vi "Main UI.vi"() -> ()   [LabVIEW 2011]
doc: "This template is for the Queued Message Handler design pattern.\n\nThe Event Handling Loop generates messages based on user interface actions.\n\nThe Message Handling Loop processes messages generated by the Event Handling Loop, or by other messages. The messages are string values, so new messages can be added easily to the Message Cases case structure in the Message Handling Loop. Each message cluster can also provide an optional value for Message Data, which is a variant that can be converted to whatever message-specific data is required."
uses:
  controls/UI Data.ctl
  support/Message Queue/Message Queue.lvlib
  support/User Event - Stop/User Event - Stop.lvlib
panel:
  out "DNL_Data Display <Replace Me>":string
  in  "DNL_Do Something Else <Replace Me>":bool
  in  "DNL_Do Something <Replace Me>":bool
  in  "DNL_Stop Button":bool
  # "These controls have associated \"Value Changed\" events configured in the Event Structure on the diagram.\n\nReplace them (and reconfigure the Event Structure) with the controls you need for your application."
  # "This template is for the Queued Message Handler design pattern.\n\nSee the block diagram for more information on how to use this template."
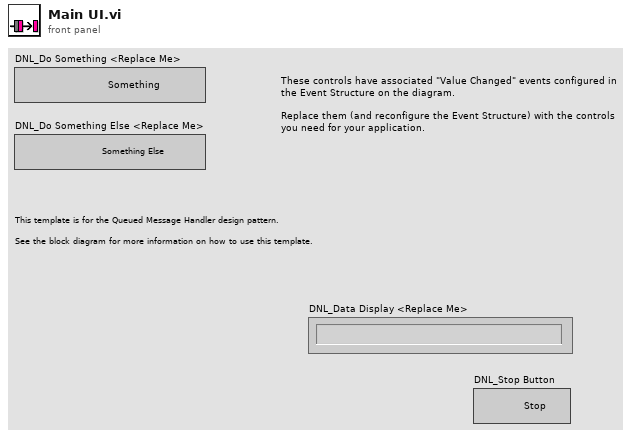
[diagram p1: front panel]
types:
  T1 = typedef "UI Data.ctl" = cluster{"DNL_Boolean <Replace Me>":bool, "DNL_String <Replace Me>":string, "DNL_Numeric <Replace Me>":dbl}
  T2 = typedef "Message Queue.lvlib/All Message Queues.ctl" = cluster{"DNL_UI":refnum<queue>}
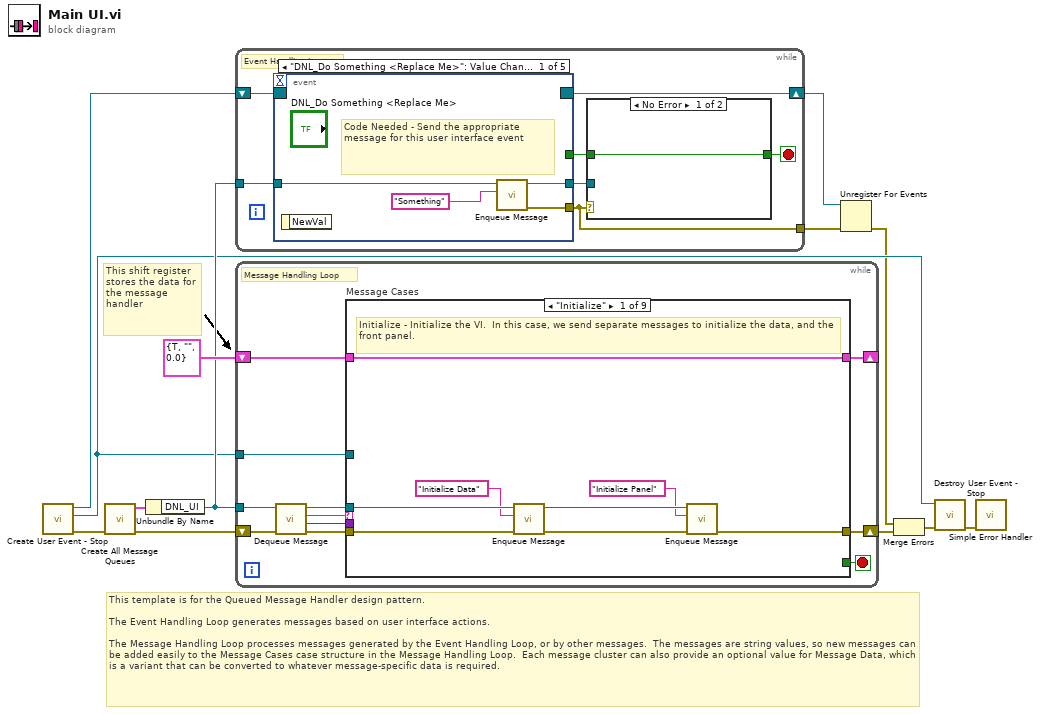
[diagram p0: block diagram]
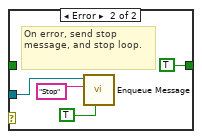
[diagram p2: hidden frame]
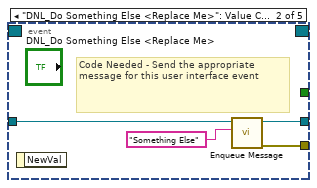
[diagram p3: hidden frame]
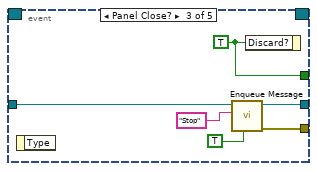
[diagram p4: hidden frame]
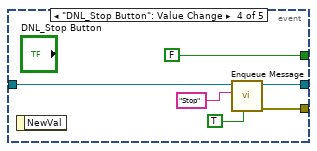
[diagram p5: hidden frame]
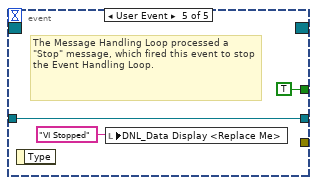
[diagram p6: hidden frame]
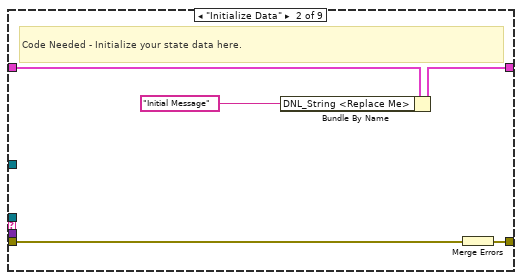
[diagram p7: hidden frame]
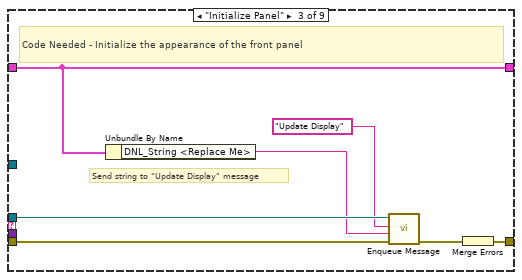
[diagram p8: hidden frame]
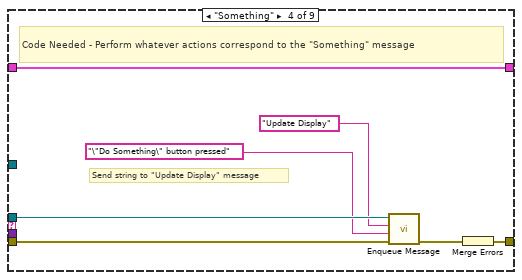
[diagram p9: hidden frame]
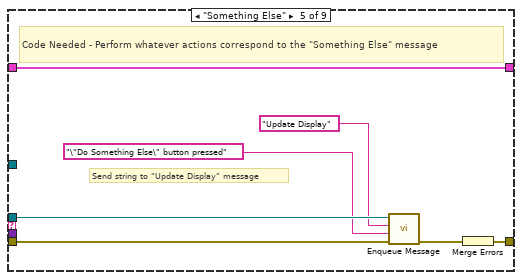
[diagram p10: hidden frame]
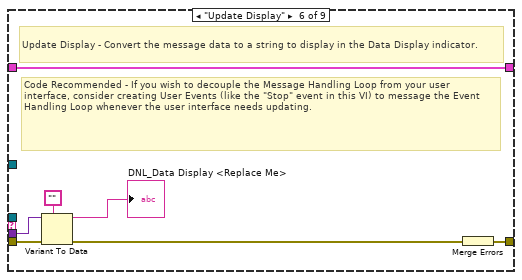
[diagram p11: hidden frame]
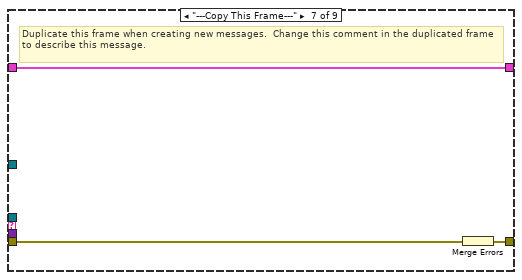
[diagram p12: hidden frame]
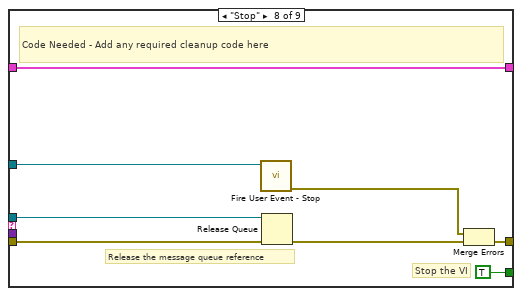
[diagram p13: hidden frame]
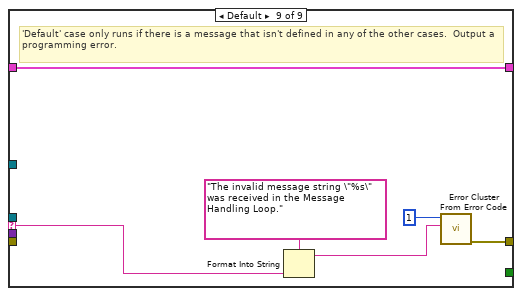
[diagram p14: hidden frame]
diagram:
  # "This template is for the Queued Message Handler design pattern.\n\nThe Event Handling Loop generates messages based on user interface actions.\n\nThe Message Handling Loop processes messages generated by the Event Handling Loop, or by other messages.  The messages are string values, so new messages can be added easily to the Message Cases case structure in the Message Handling Loop.  Each message cluster can also provide an optional value for Message Data, which is a variant that can be converted to whatever message-specific data is required."
  # "This shift register\nstores the data for the message handler"
  n1 = call "Create User Event - Stop.vi"() -> ("error out"=w7:errorcluster, "DNL_User Event - Stop"=w4:refnum<user-event>, "DNL_Stop Event Registration Refnum"=w8:refnum<event-registration>)  [unwired: 9 in]
  n2 = call "Create All Message Queues.vi"("error in (no error)"=w7) -> ("error out"=w13:errorcluster, "DNL_Message Queues out"=w11:T2)  [unwired: 9 in]
  n3 = Unbundle By Name(w11) -> ("DNL_UI"=w9:refnum<queue>)
  n4 = while {
    tunnel: w9 -> [w20]
    tunnel: [w16] -> w2
    shift-right: [w14] -> w1
    shift-left: w8 -> [w15]
    stop <- w18 stop-if-true
    # "Event Handling Loop"
    n5 = event shown="[0] \"DNL_Do Something <Replace Me>\": Value Change" {
      selector: w15 -> [_ _ _ _ _]
      dyn-events: [_ _ _ _ _] -> w14
      timeout: _ -> [_ _ _ _ _]
      tunnel: [_ _ w39 FALSE ("Discard?") TRUE ("Discard?")] -> w19
      tunnel: w20 -> [w29 w33 w38 w45 w48]
      tunnel: [w28 w31 w37 w44 _] -> w16
      tunnel: [w27 w32 w36 w42 w48] -> w17
      event "DNL_Do Something <Replace Me>": Value Change {
        # "Code Needed - Send the appropriate message for this user interface event"
        n6 = event-data() -> ()  [unwired: 1 in, 1 out]
        n7 = call "Enqueue Message.vi"("DNL_Message"="Something" ("Message"), "DNL_Message Queue"=w29) -> ("error out"=w28:errorcluster, "DNL_dup Message Queue"=w27:refnum<queue>)  [unwired: 8 in]
      }
      event "DNL_Do Something Else <Replace Me>": Value Change {
        # "Code Needed - Send the appropriate message for this user interface event"
        n8 = event-data() -> ()  [unwired: 1 in, 1 out]
        n9 = call "Enqueue Message.vi"("DNL_Message"="Something Else" ("Message"), "DNL_Message Queue"=w33) -> ("error out"=w31:errorcluster, "DNL_dup Message Queue"=w32:refnum<queue>)  [unwired: 8 in]
      }
      event Panel Close? {
        w39 = TRUE ("Discard?")
        n10 = event-data() -> ()  [unwired: 1 in, 1 out]
        n11 = call "Enqueue Message.vi"("DNL_Priority Message? (F)"=TRUE ("Priority Message? (F)"), "DNL_Message"="Stop" ("Message"), "DNL_Message Queue"=w38) -> ("error out"=w37:errorcluster, "DNL_dup Message Queue"=w36:refnum<queue>)  [unwired: 7 in]
        n12 = event-data("Discard?"=w39) -> ()  [unwired: 1 in, 1 out]
      }
      event "DNL_Stop Button": Value Change {
        n13 = event-data() -> ()  [unwired: 1 in, 1 out]
        n14 = call "Enqueue Message.vi"("DNL_Priority Message? (F)"=TRUE ("Priority Message? (F)"), "DNL_Message"="Stop" ("Message"), "DNL_Message Queue"=w45) -> ("error out"=w44:errorcluster, "DNL_dup Message Queue"=w42:refnum<queue>)  [unwired: 7 in]
      }
      event User Event {
        # "The Message Handling Loop processed a \"Stop\" message, which fired this event to stop the Event Handling Loop."
        n15 = event-data() -> ()  [unwired: 1 in, 1 out]
        n16 = local write "DNL_Data Display <Replace Me>"("VI Stopped" ("VI Stopped")) -> ()
      }
    }
    n17 = case shown="No Error" w16 {
      tunnel: [w21 TRUE ("Discard?")] -> w18
      tunnel: w19 -> [w21 _]
      tunnel: w17 -> [_ w24]
      frame No Error {
      }
      frame Error {
        # "On error, send stop message, and stop loop."
        n18 = call "Enqueue Message.vi"("DNL_Priority Message? (F)"=TRUE ("Priority Message? (F)"), "DNL_Message"="Stop" ("Message"), "DNL_Message Queue"=w24) -> ()  [unwired: 7 in, 2 out]
      }
    }
  }
  n19 = while {
    tunnel: w9 -> [w49]
    shift-right: [w58] -> _
    shift-left: T1 {"DNL_Boolean <Replace Me>"=TRUE, "DNL_String <Replace Me>"="", "DNL_Numeric <Replace Me>"=0.0} ("Data Cluster") -> [w59]
    tunnel: w4 -> [w55]
    shift-right: [w56] -> w10
    shift-left: w13 -> [w54]
    stop <- w57 stop-if-true
    # "Message Handling Loop"
    n20 = call "Dequeue Message.vi"("error in (no error)"=w54, "DNL_Message Queue"=w49) -> ("error out"=w53:errorcluster, "DNL_Message Data"=w51:variant, "DNL_Message"=w52:string, "DNL_dup Message Queue"=w50:refnum<queue>)  [unwired: 6 in]
    n21 = case "Message Cases" shown="\"Initialize\"" w52 {
      selector: w52 -> [_ _ _ _ _ _ _ _ w115]
      tunnel: w50 -> [w62 _ w76 w82 w89 _ _ w111 _]
      tunnel: w53 -> [w65 w72 w77 w84 w91 w98 w103 w106 _]
      tunnel: [w67 w68 w78 w85 w92 w99 w101 w107 w113] -> w56
      tunnel: w59 -> [w66 w71 w79 w86 w93 w100 w102 w110 w117]
      tunnel: [w66 w70 w79 w86 w93 w100 w102 w110 w117] -> w58
      tunnel: [_ _ _ _ _ _ _ TRUE _] -> w57
      tunnel: w51 -> [_ _ _ _ _ w97 _ _ _]
      tunnel: w55 -> [_ _ _ _ _ _ _ w105 _]
      frame "Initialize" {
        # "Initialize - Initialize the VI.  In this case, we send separate messages to initialize the data, and the front panel."
        n22 = call "Enqueue Message.vi"("error in (no error)"=w65, "DNL_Message"="Initialize Data" ("Message"), "DNL_Message Queue"=w62) -> ("error out"=w64:errorcluster, "DNL_dup Message Queue"=w63:refnum<queue>)  [unwired: 7 in]
        n23 = call "Enqueue Message.vi"("error in (no error)"=w64, "DNL_Message"="Initialize Panel" ("Message"), "DNL_Message Queue"=w63) -> ("error out"=w67:errorcluster)  [unwired: 7 in, 1 out]
      }
      frame "Initialize Data" {
        # "Code Needed - Initialize your state data here."
        n24 = Bundle By Name(cluster=w71, "DNL_String <Replace Me>"="Initial Message" ("Initial Message")) -> (w70:T1)
        n25 = Merge Errors(w72) -> (w68:errorcluster)
      }
      frame "Initialize Panel" {
        # "Send string to \"Update Display\" message"
        # "Code Needed - Initialize the appearance of the front panel"
        n26 = Unbundle By Name(w79) -> ("DNL_String <Replace Me>"=w73:string)
        n27 = call "Enqueue Message.vi"("error in (no error)"=w77, "DNL_Message Data"=w73, "DNL_Message"="Update Display" ("Message"), "DNL_Message Queue"=w76) -> ("error out"=w75:errorcluster)  [unwired: 6 in, 1 out]
        n28 = Merge Errors(w75) -> (w78:errorcluster)
      }
      frame "Something" {
        # "Send string to \"Update Display\" message"
        # "Code Needed - Perform whatever actions correspond to the \"Something\" message"
        n29 = call "Enqueue Message.vi"("error in (no error)"=w84, "DNL_Message Data"="\"Do Something\" button pressed" ("\"Do Something\" button pressed"), "DNL_Message"="Update Display" ("Message"), "DNL_Message Queue"=w82) -> ("error out"=w83:errorcluster)  [unwired: 6 in, 1 out]
        n30 = Merge Errors(w83) -> (w85:errorcluster)
      }
      frame "Something Else" {
        # "Send string to \"Update Display\" message"
        # "Code Needed - Perform whatever actions correspond to the \"Something Else\" message"
        n31 = call "Enqueue Message.vi"("error in (no error)"=w91, "DNL_Message Data"="\"Do Something Else\" button pressed" ("\"Do Something Else\" button pressed"), "DNL_Message"="Update Display" ("Message"), "DNL_Message Queue"=w89) -> ("error out"=w90:errorcluster)  [unwired: 6 in, 1 out]
        n32 = Merge Errors(w90) -> (w92:errorcluster)
      }
      frame "Update Display" {
        # "Code Recommended - If you wish to decouple the Message Handling Loop from your user interface, consider creating User Events (like the \"Stop\" event in this VI) to message the Event Handling Loop whenever the user interface needs updating."
        # "Update Display - Convert the message data to a string to display in the Data Display indicator."
        n33 = Variant To Data(error in=w98, type="", Variant=w97) -> (data=→"DNL_Data Display <Replace Me>":string, error out=w95:errorcluster)
        n34 = Merge Errors(w95) -> (w99:errorcluster)
      }
      frame "---Copy This Frame---" {
        # "Duplicate this frame when creating new messages.  Change this comment in the duplicated frame to describe this message."
        n35 = Merge Errors(w103) -> (w101:errorcluster)
      }
      frame "Stop" {
        # "Stop the VI"
        # "Release the message queue reference"
        # "Code Needed - Add any required cleanup code here"
        n36 = call "Fire User Event - Stop.vi"("DNL_User Event - Stop"=w105) -> ("error out"=w104:errorcluster)  [unwired: 10 in]
        n37 = Release Queue(queue=w111, error in (no error)=w106) -> (error out=w108:errorcluster)  [unwired: 1 in, 2 out]
        n38 = Merge Errors(w104, w108) -> (w107:errorcluster)
      }
      frame Default {
        # "'Default' case only runs if there is a message that isn't defined in any of the other cases.  Output a programming error."
        n39 = Format Into String(format string="The invalid message string \"%s\" was received in the Message Handling Loop." ("Unknown Message Error Text"), w115) -> (resulting string=w112:string)  [unwired: 2 in, 1 out]
        n40 = call <vilib>:"Error Cluster From Error Code.vi"("error message (\"\")"=w112, "error code (0)"=1) -> ("error out"=w113:errorcluster)  [unwired: 7 in]
      }
    }
  }
  n41 = Unregister For Events(event registration refnum=w1, error in=w2) -> (error out=w3:errorcluster)
  n42 = Merge Errors(w3, w10) -> (w5:errorcluster)
  n43 = call "Destroy User Event - Stop.vi"("error in (no error)"=w5, "DNL_User Event - Stop"=w4) -> ("error out"=w6:errorcluster)  [unwired: 9 in]
  n44 = call <vilib>:"Simple Error Handler.vi"("error in (no error)"=w6) -> ()  [unwired: 4 in, 5 out]
